vi "Conbasemela.vi"() -> ()   [LabVIEW 2020]
uses:
  PAGINAS.ctl
  <vilib>/Utility/NIReport.llb/Report Type.ctl
  <vilib>/addons/_office/excel.llb/Excel Get Data ([str]).vi
  <vilib>/Utility/NIReport.llb/Append Text Table to Report (wrap).vi
  <vilib>/regexp/Match Regular Expression.xnode
  <vilib>/Utility/NIReport.llb/NI_report.lvclass
  <vilib>/Utility/NIReport.llb/Excel/NI_Excel.lvclass
  <vilib>/Utility/NIReport.llb/NI_ReportGenerationCore.lvlib
  <vilib>/addons/_office/NI_ReportGenerationToolkit.lvlib
panel:
  in  "Sesion Iniciada TAB2":string[](array[string])
  in  "Sesion Iniciada TAB1":string[](array[string])
  in  "Tab Control 2":enum32{"LOGIN", "ADMIN", "USUARIO"}(tab)
  in  "INGRESAR 2":bool
  in  "Usuario 2":string
  in  "Contraseña 2":string
  in  "Pass add/elim 2":string
  in  "User add/elim 2":string
  in  "Terminar sesion admin 2":bool=TRUE
  in  "Añadir usuario 2":bool=TRUE
  in  "Eliminar usuario 2":bool=TRUE
  out "Dados de alta 2":string[](array[string])
  in  "Terminar sesion 2":bool=TRUE
  out "String 2":string="Hola"
  in  "MS Office parameters 2":T1={"position (excel)"={"row"=0, "column"=1}, "name (excel)"="", "bookmark (word)"=""}
  in  "MS Office parameters":T1={"position (excel)"={"row"=0, "column"=1}, "name (excel)"="", "bookmark (word)"=""}
  out "usupass juntos":string[][](array[string])
  out "data":string[][](array[string])
  in  "Pass":string[](array[string])
  in  "Usu":string[](array[string])
  in  "Tab Control":enum32{"LOGIN", "ADMIN", "USUARIO"}(tab)
  in  "INGRESAR":bool
  in  "Usuario":string
  in  "Contraseña":string
  in  "Pass add/elim":string
  in  "User add/elim":string
  in  "Terminar sesion admin":bool=TRUE
  in  "Añadir usuario":bool=TRUE
  in  "Eliminar usuario":bool=TRUE
  out "Dados de alta":string[](array[string])
  in  "Terminar sesion":bool=TRUE
  out "String":string="Hola"
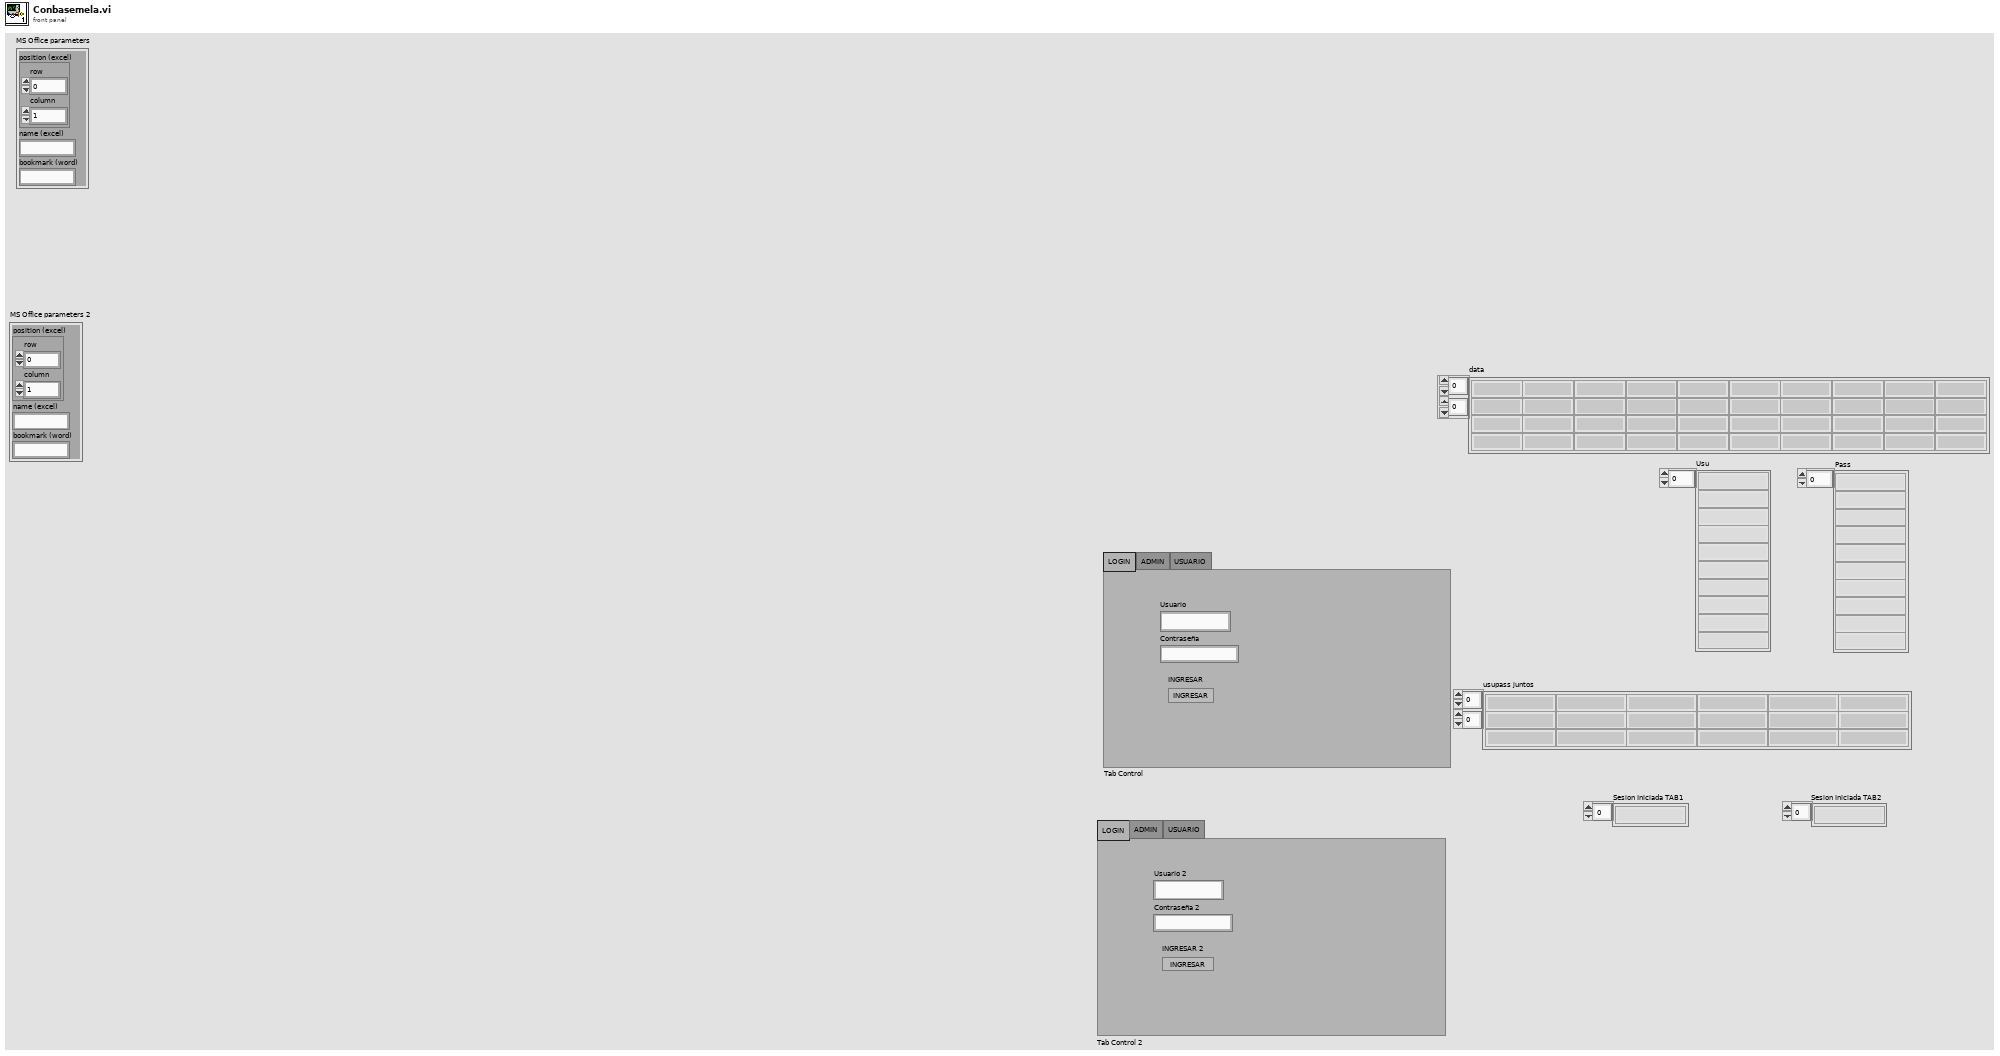
[diagram p1: front panel]
types:
  T1 = cluster{"position (excel)":cluster{"row":i32, "column":i32}, "name (excel)":string, "bookmark (word)":string}
  T2 = typedef "PAGINAS.ctl" = enum16{"0", "1", "2", "3"}
  T3 = typedef "NI_ReportGenerationCore.lvlib/Report Type.ctl" = enum16{"HTML", "Word", "Excel"}
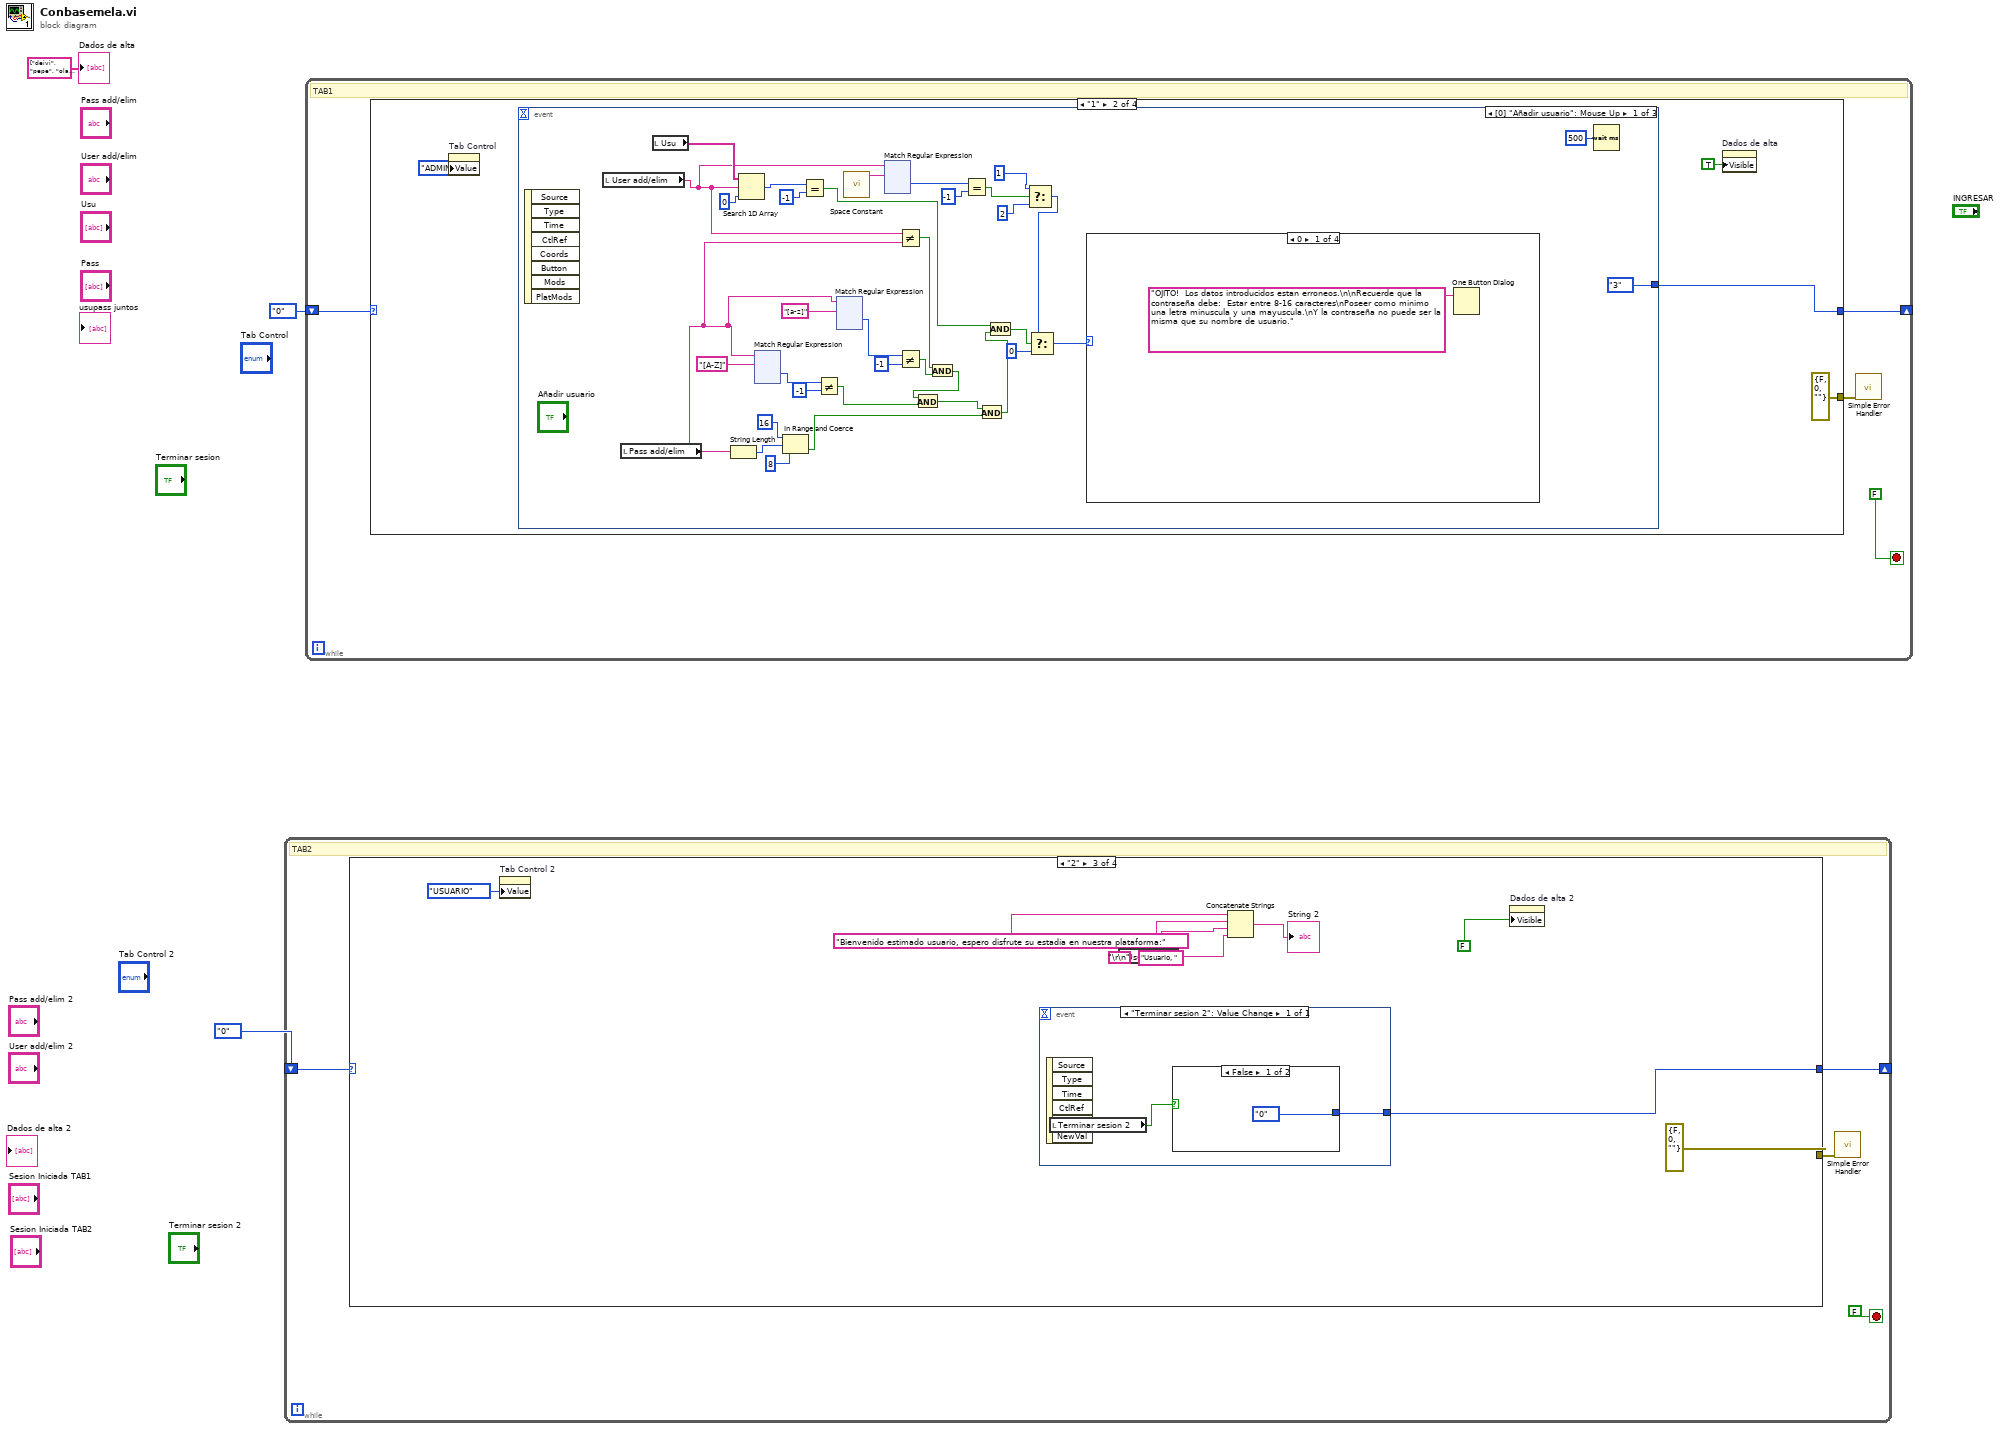
[diagram p0: block diagram]
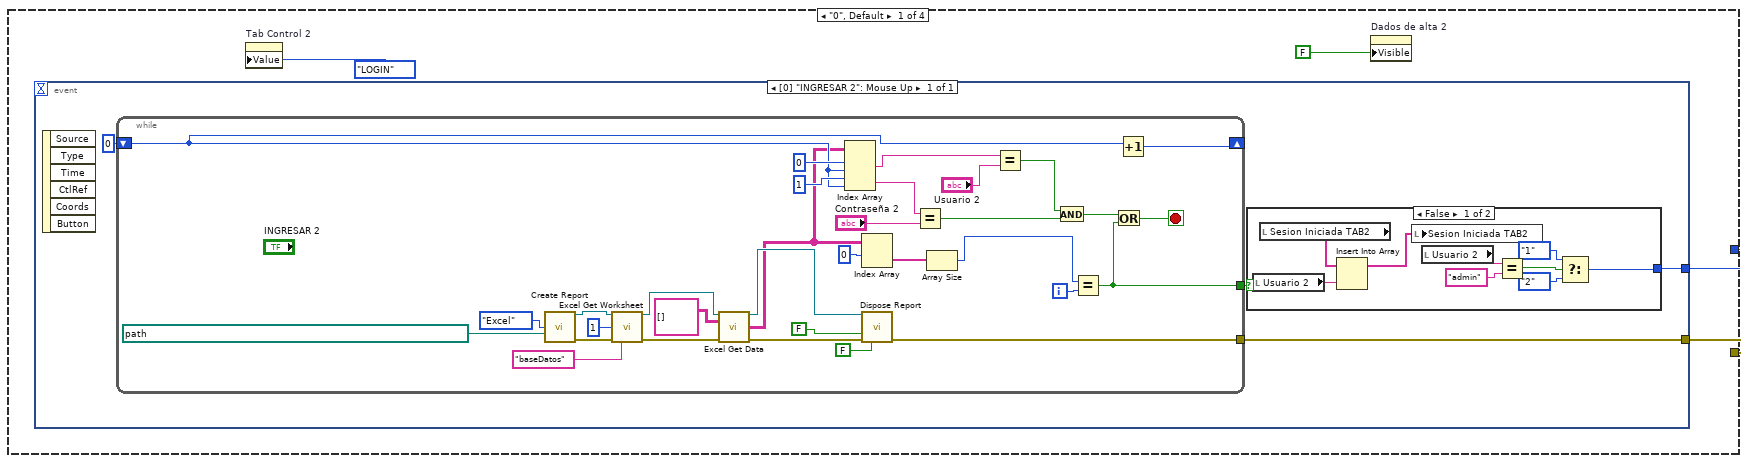
[diagram p2: hidden frame]
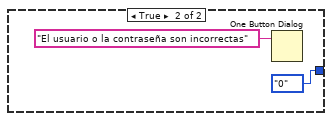
[diagram p3: hidden frame]
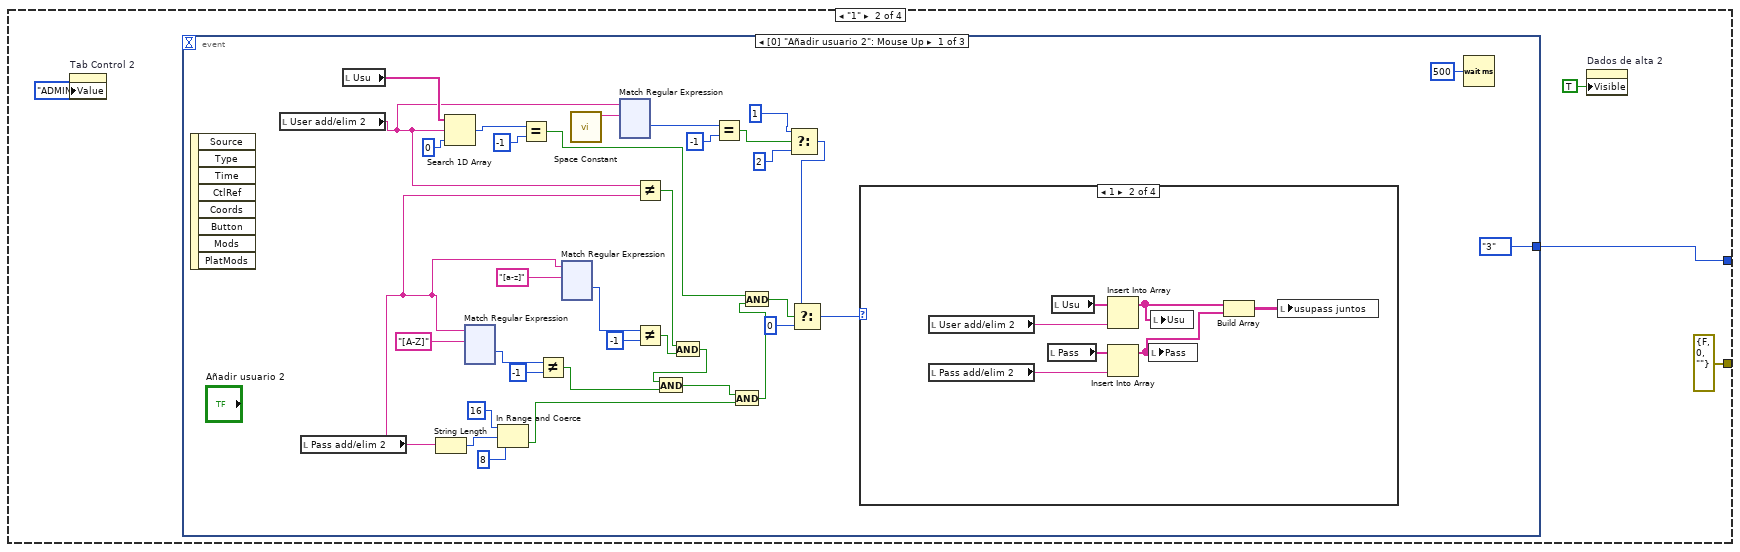
[diagram p4: hidden frame]
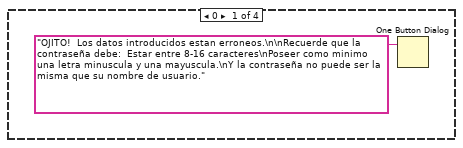
[diagram p5: hidden frame]
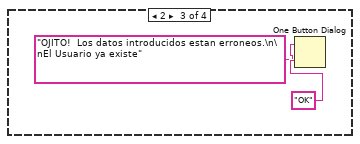
[diagram p6: hidden frame]
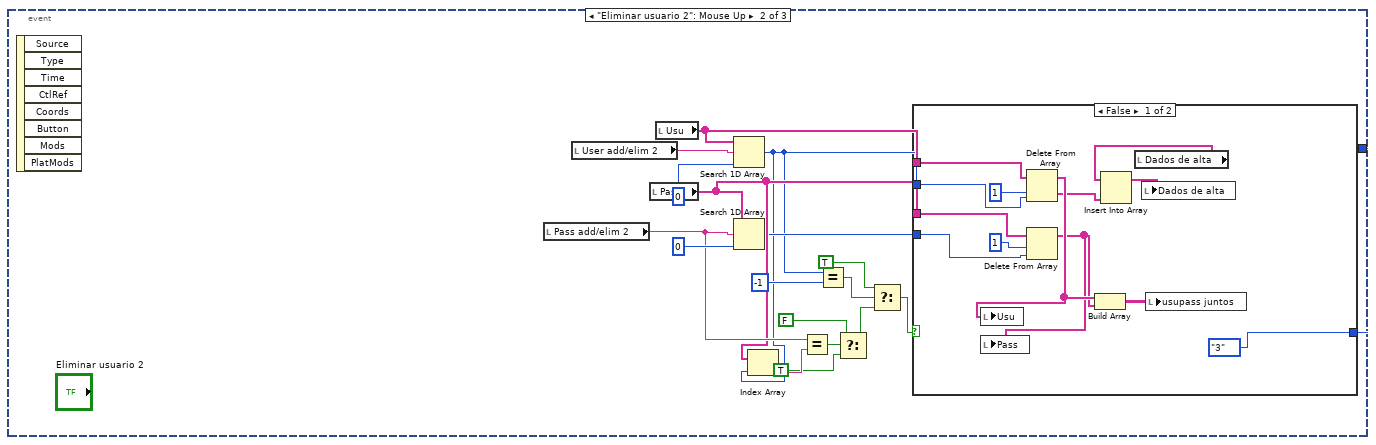
[diagram p8: hidden frame]
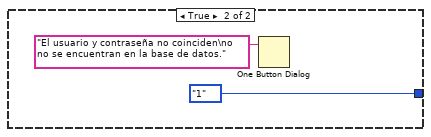
[diagram p9: hidden frame]
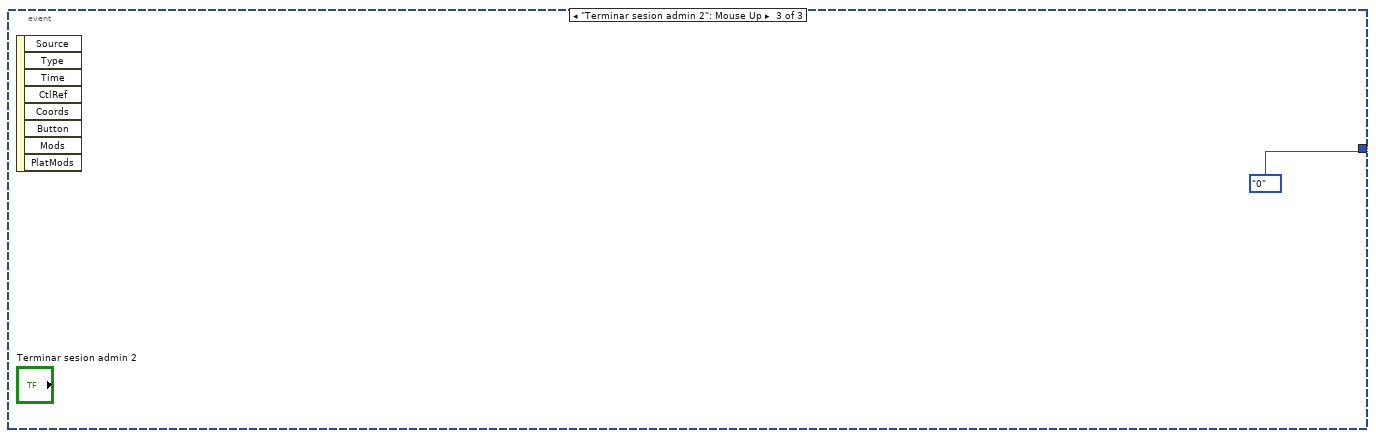
[diagram p10: hidden frame]
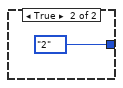
[diagram p11: hidden frame]
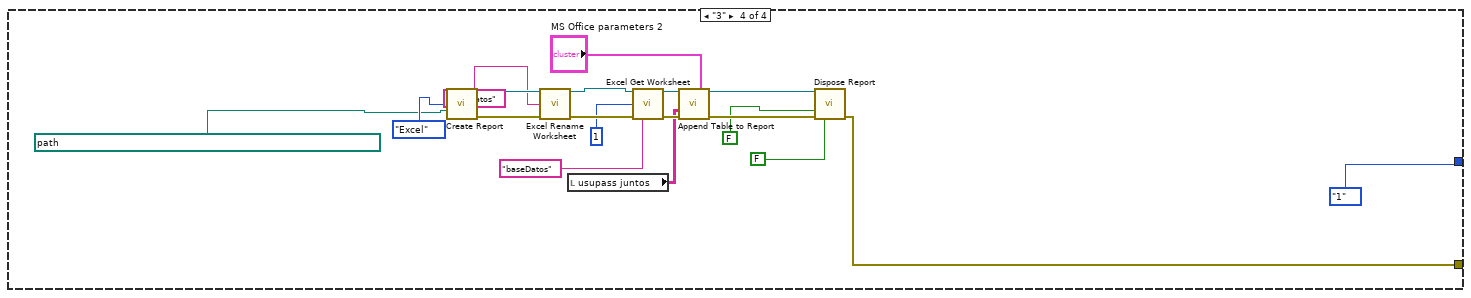
[diagram p12: hidden frame]
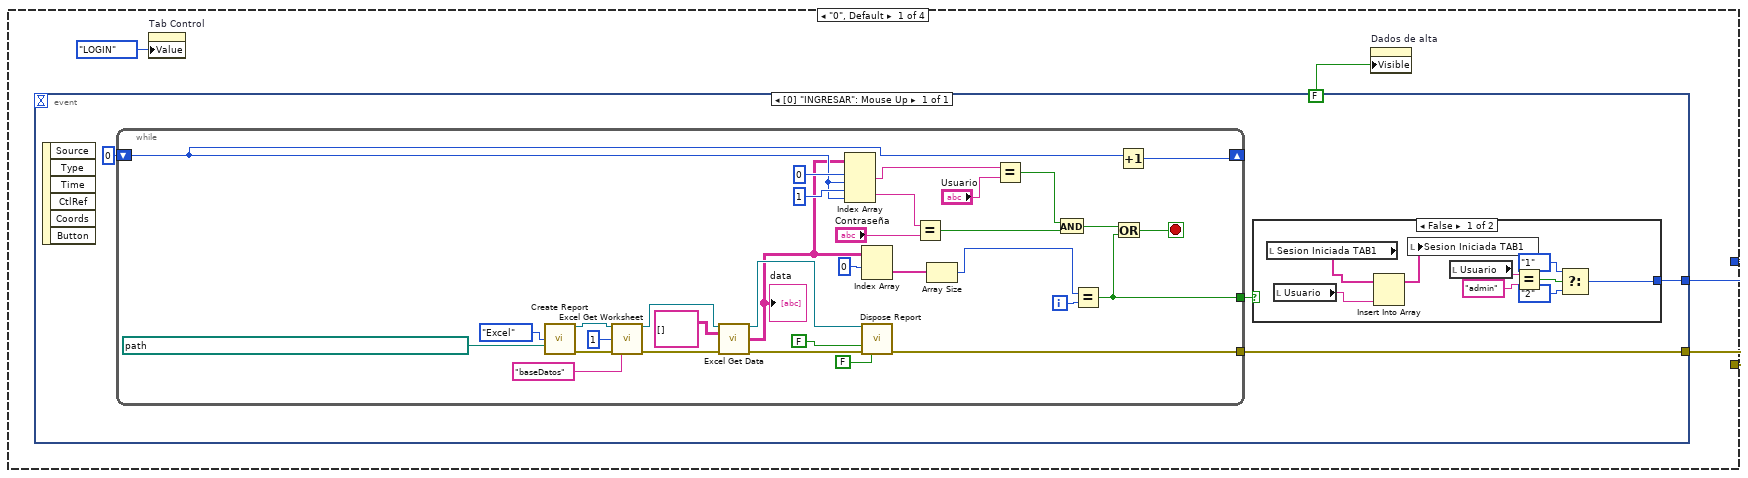
[diagram p13: hidden frame]
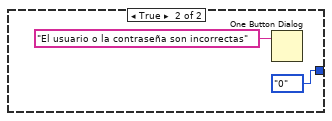
[diagram p14: hidden frame]
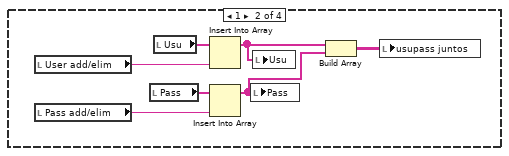
[diagram p15: hidden frame]
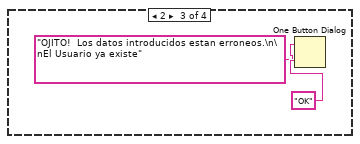
[diagram p16: hidden frame]
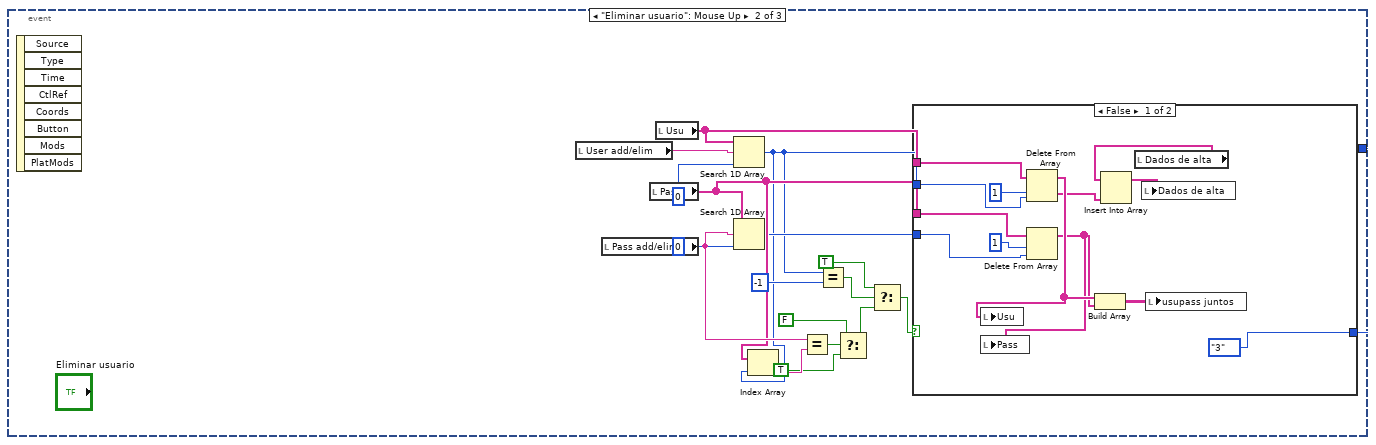
[diagram p18: hidden frame]
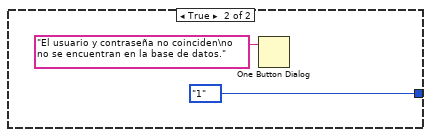
[diagram p19: hidden frame]
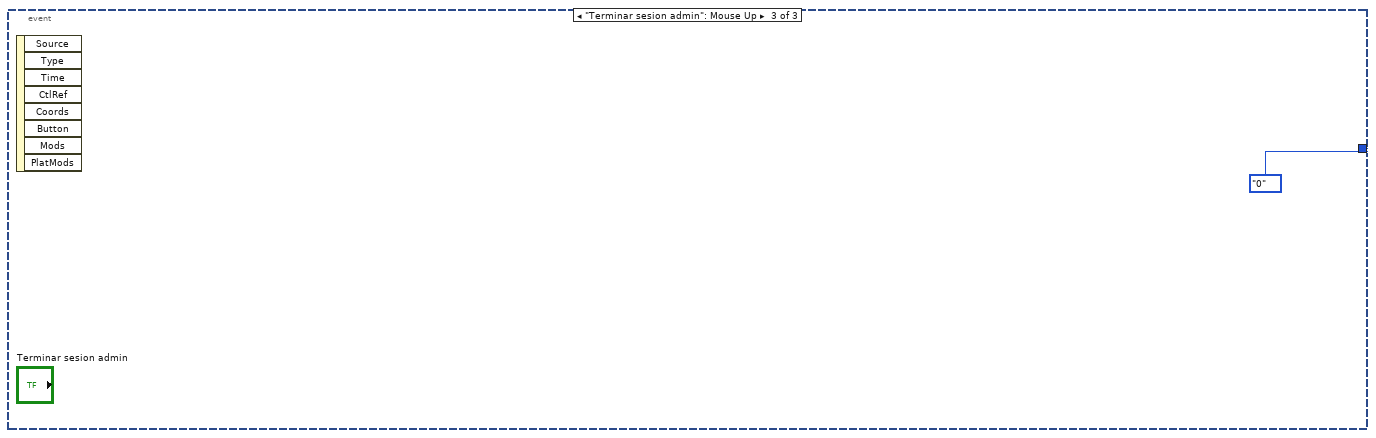
[diagram p20: hidden frame]
diagram:
  n1 = while {
    shift-right: [w6] -> _
    shift-left: PAGINAS."0" ("Enum") -> [w7]
    stop <- FALSE stop-if-true
    # "TAB2"
    n2 = case shown="\"2\"" w7 {
      tunnel: [w10 w61 w484 PAGINAS."1" ("Enum")] -> w6
      tunnel: [w9 errorcluster {"status"=FALSE, "code"=0, "source"=""} ("error out") errorcluster {"status"=FALSE, "code"=0, "source"=""} ("error out") w498] -> w4
      frame "0", Default {
        n3 = event shown="[0] \"INGRESAR 2\": Mouse Up" {
          selector: _ -> [_]
          dyn-events: _ -> [_]
          timeout: _ -> [_]
          tunnel: [w13] -> w10
          tunnel: [w12] -> w9
          event "INGRESAR 2": Mouse Up {
            n4 = event-data() -> ()  [unwired: 1 in, 6 out]
            n5 = while {
              shift-right: [w46] -> _
              shift-left: 0 -> [w39]
              tunnel: [w28] -> w14
              tunnel: [w27] -> w12
              i -> [w32]
              stop <- w29 stop-if-true
              n6 = call <vilib>:"Create Report.vi"("report type"=Report_Type."Excel", "template (empty)"=path "E:/2020-2/Lenguaje de programación ll/quiz 3.1/baseDatos.xlsx" ("file path (dialog if empty)")) -> ("report out"=w56:refnum<class "NI_report.lvclass">, "error out"=w55:errorcluster)  [unwired: 12 in]
              n7 = call <vilib>:"Excel Get Worksheet.vi"("report in"=w56, "worksheet index (0)"=1, "error in (no error)"=w55, "name (\"\")"="baseDatos" ("name (\"\")")) -> ("report out"=w53:refnum<class "NI_report.lvclass">, "error out"=w52:errorcluster)  [unwired: 10 in]
              n8 = call-poly <vilib>:"Excel Get Data.vi"("report in"=w53, "data type"=string[][] [], "error in (no error)"=w52) -> ("report out"=w51:refnum<class "NI_report.lvclass">, "data"=w35:string[][], "error out"=w50:errorcluster)  [unwired: 10 in]
              n9 = Index Array(array=w35, index (row) #1=0 ("index (row)"), index (col) #1=w39, index (row) #2=1 ("index (row)"), index (col) #2=w39) -> (element #1=w45:string, element #2=w38:string)
              n10 = Index Array(array=w35, index (row)=0) -> (element=w33:string[])  [unwired: 1 in]
              n11 = call-dynamic "Dispose Report.vi"("report in"=w51, "save changes? (F)"=FALSE, "error in (no error)"=w50, "close report? (T)"=FALSE) -> ("error out"=w27:errorcluster)  [unwired: 11 in]
              n12 = Equal?(x=w38, y="Contraseña 2") -> (x = y?=w42:bool)
              n13 = Array Size(array=w33) -> (size(s)=w31:i32)
              n14 = Equal?(x=w45, y="Usuario 2") -> (x = y?=w43:bool)
              n15 = And(x=w43, y=w42) -> (x .and. y?=w30:bool)
              n16 = Equal?(x=w31, y=w32) -> (x = y?=w28:bool)
              n17 = Or(x=w30, y=w28) -> (x .or. y?=w29:bool)
              n18 = Increment(x=w39) -> (x+1=w46:i32)
            }
            n19 = case shown="False" w14 {
              tunnel: [w19 PAGINAS."0" ("Enum")] -> w13
              frame False {
                n20 = local read "Usuario 2"() -> (w18:string)
                n21 = local read "Sesion Iniciada TAB2"() -> (w16:string[])
                n22 = Insert Into Array(array=w16, new element=w18) -> (w17:string[])  [unwired: 1 in]
                n23 = local write "Sesion Iniciada TAB2"(w17) -> ()
                n24 = local read "Usuario 2"() -> (w23:string)
                n25 = Equal?(x=w23, y="admin") -> (x = y?=w24:bool)
                n26 = Select(t=PAGINAS."1" ("Enum"), s=w24, f=PAGINAS."2" ("Enum")) -> (s? t:f=w19:T2)
              }
              frame True {
                n27 = One Button Dialog(message="El usuario o la contraseña son incorrectas") -> ()  [unwired: 1 in, 1 out]
              }
            }
          }
        }
        n28 = property on="Tab Control 2" class="TabCtl (strict)"("Value"=enum32{"LOGIN", "ADMIN", "USUARIO"}."LOGIN" ("Tab Control")) -> ()  [unwired: 2 in, 2 out]
        n29 = property on="Dados de alta 2" class="Arr (strict)"("Visible"=FALSE) -> ()  [unwired: 2 in, 2 out]
      }
      frame "1" {
        n30 = property on="Tab Control 2" class="TabCtl (strict)"("Value"=enum32{"LOGIN", "ADMIN", "USUARIO"}."ADMIN" ("Tab Control")) -> ()  [unwired: 2 in, 2 out]
        n31 = event shown="[0] \"Añadir usuario 2\": Mouse Up" {
          selector: _ -> [_ _ _]
          dyn-events: _ -> [_ _ _]
          timeout: _ -> [_ _ _]
          tunnel: [PAGINAS."3" ("Enum") w463 PAGINAS."0" ("Enum")] -> w61
          event "Añadir usuario 2": Mouse Up {
            n32 = event-data() -> ()  [unwired: 1 in, 8 out]
            n33 = local read "User add/elim 2"() -> (w75:string)
            n34 = local read "Pass add/elim 2"() -> (w79:string)
            n35 = local read "Usu"() -> (w96:string[])
            n36 = String Length(string=w79) -> (length=w92:i32)
            n37 = Search 1D Array(1D array=w96, element=w75, start index (0)=0) -> (index of element=w94:i32)
            n38 = xnode "Match Regular Expression"("input string"=w79, "regular expression"="[A-Z]") -> ("offset past match"=w88:i32)  [unwired: 4 in, 4 out]
            n39 = In Range and Coerce(upper limit=16, x=w92, lower limit=8) -> (In Range?=w77:bool)  [unwired: 1 out]
            n40 = Equal?(x=w94, y=-1) -> (x = y?=w71:bool)
            n41 = Not Equal?(x=w88, y=-1) -> (x != y?=w80:bool)
            n42 = xnode "Match Regular Expression"("input string"=w79, "regular expression"="[a-z]") -> ("offset past match"=w84:i32)  [unwired: 4 in, 4 out]
            n43 = call <vilib>:"Space Constant.vi"() -> ("String"=w74:string)
            n44 = xnode "Match Regular Expression"("input string"=w75, "regular expression"=w74) -> ("offset past match"=w72:i32)  [unwired: 4 in, 4 out]
            n45 = Not Equal?(x=w75, y=w79) -> (x != y?=w78:bool)
            n46 = Not Equal?(x=w84, y=-1) -> (x != y?=w82:bool)
            n47 = And(x=w78, y=w82) -> (x .and. y?=w81:bool)
            n48 = And(x=w81, y=w80) -> (x .and. y?=w76:bool)
            n49 = Equal?(x=w72, y=-1) -> (x = y?=w69:bool)
            n50 = And(x=w76, y=w77) -> (x .and. y?=w70:bool)
            n51 = And(x=w71, y=w70) -> (x .and. y?=w67:bool)
            n52 = Select(t=1 ("y"), s=w69, f=2 ("y")) -> (s? t:f=w66:i32)
            n53 = Select(t=w66, s=w67, f=0) -> (s? t:f=w65:i32)
            n54 = case shown="1" w65 {
              frame 0 {
                n55 = One Button Dialog(message="OJITO!  Los datos introducidos estan erroneos.\n\nRecuerde que la contraseña debe:  Estar entre 8-16 caracteres\nPoseer como minimo una letra minuscula y una mayuscula.\nY la contraseña no puede ser la misma que su nombre de usuario.") -> ()  [unwired: 1 in, 1 out]
              }
              frame 1 {
                n56 = local read "User add/elim 2"() -> (w216:string)
                n57 = local read "Pass add/elim 2"() -> (w217:string)
                n58 = local read "Pass"() -> (w218:string[])
                n59 = local read "Usu"() -> (w219:string[])
                n60 = Insert Into Array(array=w219, new element=w216) -> (w215:string[])  [unwired: 1 in]
                n61 = Insert Into Array(array=w218, new element=w217) -> (w214:string[])  [unwired: 1 in]
                n62 = local write "Pass"(w214) -> ()
                n63 = local write "Usu"(w215) -> ()
                n64 = Build Array(w215, w214) -> (w213:string[][])
                n65 = local write "usupass juntos"(w213) -> ()
              }
              frame 2 {
                n66 = One Button Dialog(message="OJITO!  Los datos introducidos estan erroneos.\n\nEl Usuario ya existe", button name ("OK")="OK") -> ()  [unwired: 1 out]
              }
              frame 3, Default {
              }
            }
            n67 = Wait (ms)(milliseconds to wait=u32 500) -> ()  [unwired: 1 out]
          }
          event "Eliminar usuario 2": Mouse Up {
            n68 = event-data() -> ()  [unwired: 1 in, 8 out]
            n69 = local read "Pass add/elim 2"() -> (w461:string)
            n70 = local read "User add/elim 2"() -> (w467:string)
            n71 = local read "Pass"() -> (w453:string[])
            n72 = local read "Usu"() -> (w451:string[])
            n73 = Search 1D Array(1D array=w451, element=w467, start index (0)=0) -> (index of element=w450:i32)
            n74 = Search 1D Array(1D array=w453, element=w461, start index (0)=0) -> (index of element=w452:i32)
            n75 = Index Array(array=w453, index=w450) -> (element=w462:string)
            n76 = Equal?(x=w461, y=w462) -> (x = y?=w457:bool)
            n77 = Equal?(x=w450, y=-1) -> (x = y?=w460:bool)
            n78 = Select(t=FALSE, s=w457, f=TRUE) -> (s? t:f=w454:bool)
            n79 = Select(t=TRUE, s=w460, f=w454) -> (s? t:f=w458:bool)
            n80 = case shown="False" w458 {
              tunnel: [PAGINAS."3" ("Enum") PAGINAS."1" ("Enum")] -> w463
              tunnel: w453 -> [w479 _]
              tunnel: w452 -> [w477 _]
              tunnel: w451 -> [w476 _]
              tunnel: w450 -> [w474 _]
              frame False {
                n81 = Delete From Array(array=w476, length=1, index=w474) -> (deleted portion=w469:string[], array with subset deleted=w472:string[])
                n82 = local write "Usu"(w472) -> ()
                n83 = Delete From Array(array=w479, length=1, index=w477) -> (array with subset deleted=w471:string[])  [unwired: 1 out]
                n84 = local write "Pass"(w471) -> ()
                n85 = Build Array(w472, w471) -> (w473:string[][])
                n86 = local read "Dados de alta"() -> (w470:string[])
                n87 = Insert Into Array(array=w470, new element=w469) -> (w468:string[])  [unwired: 1 in]
                n88 = local write "Dados de alta"(w468) -> ()
                n89 = local write "usupass juntos"(w473) -> ()
              }
              frame True {
                n90 = One Button Dialog(message="El usuario y contraseña no coinciden\no no se encuentran en la base de datos.") -> ()  [unwired: 1 in, 1 out]
              }
            }
          }
          event "Terminar sesion admin 2": Mouse Up {
            n91 = event-data() -> ()  [unwired: 1 in, 8 out]
          }
        }
        n92 = property on="Dados de alta 2" class="Arr (strict)"("Visible"=TRUE) -> ()  [unwired: 2 in, 2 out]
      }
      frame "2" {
        n93 = property on="Tab Control 2" class="TabCtl (strict)"("Value"=enum32{"LOGIN", "ADMIN", "USUARIO"}."USUARIO" ("Tab Control")) -> ()  [unwired: 2 in, 2 out]
        n94 = event shown="[0] \"Terminar sesion 2\": Value Change" {
          selector: _ -> [_]
          dyn-events: _ -> [_]
          timeout: _ -> [_]
          tunnel: [w493] -> w484
          event "Terminar sesion 2": Value Change {
            n95 = event-data() -> ()  [unwired: 1 in, 6 out]
            n96 = local read "Terminar sesion 2"() -> (w494:bool)
            n97 = case shown="False" w494 {
              tunnel: [PAGINAS."0" ("Enum") PAGINAS."2" ("Enum")] -> w493
              frame False {
              }
              frame True {
              }
            }
          }
        }
        n98 = local read "Usuario 2"() -> (w486:string)
        n99 = Concatenate Strings("Bienvenido estimado usuario, espero disfrute su estadía en nuestra plataforma:" ("string"), "\r\n", "Usuario, " ("string"), w486) -> (→"String 2":string)
        n100 = property on="Dados de alta 2" class="Arr (strict)"("Visible"=FALSE) -> ()  [unwired: 2 in, 2 out]
      }
      frame "3" {
        n101 = call <vilib>:"Create Report.vi"("report type"=Report_Type."Excel", "template (empty)"=path "E:/2020-2/Lenguaje de programación ll/quiz 3.1/baseDatos.xlsx" ("file path (dialog if empty)")) -> ("report out"=w513:refnum<class "NI_report.lvclass">, "error out"=w514:errorcluster)  [unwired: 12 in]
        n102 = call <vilib>:"Excel Rename Worksheet.vi"("report in"=w513, "worksheet name (\"\")"="baseDatos" ("worksheet name (\"\")"), "error in (no error)"=w514) -> ("report out"=w512:refnum<class "NI_report.lvclass">, "error out"=w515:errorcluster)  [unwired: 11 in]
        n103 = local read "usupass juntos"() -> (w497:string[][])
        n104 = call <vilib>:"Excel Get Worksheet.vi"("report in"=w512, "worksheet index (0)"=1, "error in (no error)"=w515, "name (\"\")"="baseDatos" ("name (\"\")")) -> ("report out"=w510:refnum<class "NI_report.lvclass">, "error out"=w509:errorcluster)  [unwired: 10 in]
        n105 = call-poly <vilib>:"Append Table to Report.vi"("report in"=w510, "MS Office parameters"="MS Office parameters 2", "text data"=w497, "error in (no error)"=w509) -> ("report out"=w508:refnum<class "NI_report.lvclass">, "error out"=w507:errorcluster)  [unwired: 8 in, 2 out]
        n106 = call-dynamic "Dispose Report.vi"("report in"=w508, "save changes? (F)"=FALSE, "error in (no error)"=w507, "close report? (T)"=FALSE) -> ("error out"=w498:errorcluster)  [unwired: 11 in]
      }
    }
    n107 = call <vilib>:"Simple Error Handler.vi"("error in (no error)"=w4) -> ()  [unwired: 4 in, 5 out]
  }
  n108 = while {
    shift-right: [w518] -> _
    shift-left: PAGINAS."0" ("Enum") -> [w519]
    stop <- FALSE stop-if-true
    # "TAB1"
    n109 = case shown="\"1\"" w519 {
      tunnel: [w522 w573 w996 PAGINAS."1" ("Enum")] -> w518
      tunnel: [w521 errorcluster {"status"=FALSE, "code"=0, "source"=""} ("error out") errorcluster {"status"=FALSE, "code"=0, "source"=""} ("error out") w1010] -> w516
      frame "0", Default {
        n110 = event shown="[0] \"INGRESAR\": Mouse Up" {
          selector: _ -> [_]
          dyn-events: _ -> [_]
          timeout: _ -> [_]
          tunnel: [w525] -> w522
          tunnel: [w524] -> w521
          event "INGRESAR": Mouse Up {
            n111 = event-data() -> ()  [unwired: 1 in, 6 out]
            n112 = while {
              shift-right: [w558] -> _
              shift-left: 0 -> [w551]
              tunnel: [w540] -> w526
              tunnel: [w539] -> w524
              i -> [w544]
              stop <- w541 stop-if-true
              n113 = call <vilib>:"Create Report.vi"("report type"=Report_Type."Excel", "template (empty)"=path "E:/2020-2/Lenguaje de programación ll/quiz 3.1/baseDatos.xlsx" ("file path (dialog if empty)")) -> ("report out"=w568:refnum<class "NI_report.lvclass">, "error out"=w567:errorcluster)  [unwired: 12 in]
              n114 = call <vilib>:"Excel Get Worksheet.vi"("report in"=w568, "worksheet index (0)"=1, "error in (no error)"=w567, "name (\"\")"="baseDatos" ("name (\"\")")) -> ("report out"=w565:refnum<class "NI_report.lvclass">, "error out"=w564:errorcluster)  [unwired: 10 in]
              n115 = call-poly <vilib>:"Excel Get Data.vi"("report in"=w565, "data type"=string[][] [], "error in (no error)"=w564) -> ("report out"=w563:refnum<class "NI_report.lvclass">, "data"=w547:string[][], "error out"=w562:errorcluster)  [unwired: 10 in]
              "data" <- w547
              n116 = Index Array(array=w547, index (row) #1=0 ("index (row)"), index (col) #1=w551, index (row) #2=1 ("index (row)"), index (col) #2=w551) -> (element #1=w557:string, element #2=w550:string)
              n117 = Index Array(array=w547, index (row)=0) -> (element=w545:string[])  [unwired: 1 in]
              n118 = call-dynamic "Dispose Report.vi"("report in"=w563, "save changes? (F)"=FALSE, "error in (no error)"=w562, "close report? (T)"=FALSE) -> ("error out"=w539:errorcluster)  [unwired: 11 in]
              n119 = Equal?(x=w550, y="Contraseña") -> (x = y?=w554:bool)
              n120 = Array Size(array=w545) -> (size(s)=w543:i32)
              n121 = Equal?(x=w557, y="Usuario") -> (x = y?=w555:bool)
              n122 = And(x=w555, y=w554) -> (x .and. y?=w542:bool)
              n123 = Equal?(x=w543, y=w544) -> (x = y?=w540:bool)
              n124 = Or(x=w542, y=w540) -> (x .or. y?=w541:bool)
              n125 = Increment(x=w551) -> (x+1=w558:i32)
            }
            n126 = case shown="False" w526 {
              tunnel: [w531 PAGINAS."0" ("Enum")] -> w525
              frame False {
                n127 = local read "Sesion Iniciada TAB1"() -> (w530:string[])
                n128 = local read "Usuario"() -> (w529:string)
                n129 = Insert Into Array(array=w530, new element=w529) -> (w528:string[])  [unwired: 1 in]
                n130 = local write "Sesion Iniciada TAB1"(w528) -> ()
                n131 = local read "Usuario"() -> (w535:string)
                n132 = Equal?(x=w535, y="admin") -> (x = y?=w536:bool)
                n133 = Select(t=PAGINAS."1" ("Enum"), s=w536, f=PAGINAS."2" ("Enum")) -> (s? t:f=w531:T2)
              }
              frame True {
                n134 = One Button Dialog(message="El usuario o la contraseña son incorrectas") -> ()  [unwired: 1 in, 1 out]
              }
            }
          }
        }
        n135 = property on="Tab Control" class="TabCtl (strict)"("Value"=enum32{"LOGIN", "ADMIN", "USUARIO"}."LOGIN" ("Tab Control")) -> ()  [unwired: 2 in, 2 out]
        n136 = property on="Dados de alta" class="Arr (strict)"("Visible"=FALSE) -> ()  [unwired: 2 in, 2 out]
      }
      frame "1" {
        n137 = property on="Tab Control" class="TabCtl (strict)"("Value"=enum32{"LOGIN", "ADMIN", "USUARIO"}."ADMIN" ("Tab Control")) -> ()  [unwired: 2 in, 2 out]
        n138 = event shown="[0] \"Añadir usuario\": Mouse Up" {
          selector: _ -> [_ _ _]
          dyn-events: _ -> [_ _ _]
          timeout: _ -> [_ _ _]
          tunnel: [PAGINAS."3" ("Enum") w975 PAGINAS."0" ("Enum")] -> w573
          event "Añadir usuario": Mouse Up {
            n139 = event-data() -> ()  [unwired: 1 in, 8 out]
            n140 = local read "User add/elim"() -> (w587:string)
            n141 = local read "Pass add/elim"() -> (w591:string)
            n142 = local read "Usu"() -> (w608:string[])
            n143 = String Length(string=w591) -> (length=w604:i32)
            n144 = Search 1D Array(1D array=w608, element=w587, start index (0)=0) -> (index of element=w606:i32)
            n145 = xnode "Match Regular Expression"("input string"=w591, "regular expression"="[A-Z]") -> ("offset past match"=w600:i32)  [unwired: 4 in, 4 out]
            n146 = In Range and Coerce(upper limit=16, x=w604, lower limit=8) -> (In Range?=w589:bool)  [unwired: 1 out]
            n147 = Equal?(x=w606, y=-1) -> (x = y?=w583:bool)
            n148 = Not Equal?(x=w600, y=-1) -> (x != y?=w592:bool)
            n149 = xnode "Match Regular Expression"("input string"=w591, "regular expression"="[a-z]") -> ("offset past match"=w596:i32)  [unwired: 4 in, 4 out]
            n150 = call <vilib>:"Space Constant.vi"() -> ("String"=w586:string)
            n151 = xnode "Match Regular Expression"("input string"=w587, "regular expression"=w586) -> ("offset past match"=w584:i32)  [unwired: 4 in, 4 out]
            n152 = Not Equal?(x=w587, y=w591) -> (x != y?=w590:bool)
            n153 = Not Equal?(x=w596, y=-1) -> (x != y?=w594:bool)
            n154 = And(x=w590, y=w594) -> (x .and. y?=w593:bool)
            n155 = And(x=w593, y=w592) -> (x .and. y?=w588:bool)
            n156 = Equal?(x=w584, y=-1) -> (x = y?=w581:bool)
            n157 = And(x=w588, y=w589) -> (x .and. y?=w582:bool)
            n158 = And(x=w583, y=w582) -> (x .and. y?=w579:bool)
            n159 = Select(t=1 ("y"), s=w581, f=2 ("y")) -> (s? t:f=w578:i32)
            n160 = Select(t=w578, s=w579, f=0) -> (s? t:f=w577:i32)
            n161 = case shown="0" w577 {
              frame 0 {
                n162 = One Button Dialog(message="OJITO!  Los datos introducidos estan erroneos.\n\nRecuerde que la contraseña debe:  Estar entre 8-16 caracteres\nPoseer como minimo una letra minuscula y una mayuscula.\nY la contraseña no puede ser la misma que su nombre de usuario.") -> ()  [unwired: 1 in, 1 out]
              }
              frame 1 {
                n163 = local read "User add/elim"() -> (w728:string)
                n164 = local read "Pass add/elim"() -> (w729:string)
                n165 = local read "Pass"() -> (w730:string[])
                n166 = local read "Usu"() -> (w731:string[])
                n167 = Insert Into Array(array=w731, new element=w728) -> (w727:string[])  [unwired: 1 in]
                n168 = Insert Into Array(array=w730, new element=w729) -> (w726:string[])  [unwired: 1 in]
                n169 = local write "Pass"(w726) -> ()
                n170 = local write "Usu"(w727) -> ()
                n171 = Build Array(w727, w726) -> (w725:string[][])
                n172 = local write "usupass juntos"(w725) -> ()
              }
              frame 2 {
                n173 = One Button Dialog(message="OJITO!  Los datos introducidos estan erroneos.\n\nEl Usuario ya existe", button name ("OK")="OK") -> ()  [unwired: 1 out]
              }
              frame 3, Default {
              }
            }
            n174 = Wait (ms)(milliseconds to wait=u32 500) -> ()  [unwired: 1 out]
          }
          event "Eliminar usuario": Mouse Up {
            n175 = event-data() -> ()  [unwired: 1 in, 8 out]
            n176 = local read "User add/elim"() -> (w979:string)
            n177 = local read "Pass add/elim"() -> (w973:string)
            n178 = local read "Pass"() -> (w965:string[])
            n179 = local read "Usu"() -> (w963:string[])
            n180 = Search 1D Array(1D array=w963, element=w979, start index (0)=0) -> (index of element=w962:i32)
            n181 = Search 1D Array(1D array=w965, element=w973, start index (0)=0) -> (index of element=w964:i32)
            n182 = Index Array(array=w965, index=w962) -> (element=w974:string)
            n183 = Equal?(x=w973, y=w974) -> (x = y?=w969:bool)
            n184 = Equal?(x=w962, y=-1) -> (x = y?=w972:bool)
            n185 = Select(t=FALSE, s=w969, f=TRUE) -> (s? t:f=w966:bool)
            n186 = Select(t=TRUE, s=w972, f=w966) -> (s? t:f=w970:bool)
            n187 = case shown="False" w970 {
              tunnel: [PAGINAS."3" ("Enum") PAGINAS."1" ("Enum")] -> w975
              tunnel: w965 -> [w991 _]
              tunnel: w964 -> [w989 _]
              tunnel: w963 -> [w988 _]
              tunnel: w962 -> [w986 _]
              frame False {
                n188 = Delete From Array(array=w988, length=1, index=w986) -> (deleted portion=w981:string[], array with subset deleted=w984:string[])
                n189 = local write "Usu"(w984) -> ()
                n190 = Delete From Array(array=w991, length=1, index=w989) -> (array with subset deleted=w983:string[])  [unwired: 1 out]
                n191 = local write "Pass"(w983) -> ()
                n192 = Build Array(w984, w983) -> (w985:string[][])
                n193 = local read "Dados de alta"() -> (w982:string[])
                n194 = Insert Into Array(array=w982, new element=w981) -> (w980:string[])  [unwired: 1 in]
                n195 = local write "Dados de alta"(w980) -> ()
                n196 = local write "usupass juntos"(w985) -> ()
              }
              frame True {
                n197 = One Button Dialog(message="El usuario y contraseña no coinciden\no no se encuentran en la base de datos.") -> ()  [unwired: 1 in, 1 out]
              }
            }
          }
          event "Terminar sesion admin": Mouse Up {
            n198 = event-data() -> ()  [unwired: 1 in, 8 out]
          }
        }
        n199 = property on="Dados de alta" class="Arr (strict)"("Visible"=TRUE) -> ()  [unwired: 2 in, 2 out]
      }
      frame "2" {
        n200 = property on="Tab Control" class="TabCtl (strict)"("Value"=enum32{"LOGIN", "ADMIN", "USUARIO"}."USUARIO" ("Tab Control")) -> ()  [unwired: 2 in, 2 out]
        n201 = event shown="[0] \"Terminar sesion\": Mouse Up" {
          selector: _ -> [_]
          dyn-events: _ -> [_]
          timeout: _ -> [_]
          tunnel: [w1005] -> w996
          event "Terminar sesion": Mouse Up {
            n202 = event-data() -> ()  [unwired: 1 in, 8 out]
            n203 = local read "Terminar sesion"() -> (w1006:bool)
            n204 = case shown="True" w1006 {
              tunnel: [PAGINAS."0" ("Enum") PAGINAS."2" ("Enum")] -> w1005
              frame False {
              }
              frame True {
              }
            }
          }
        }
        n205 = local read "Usuario"() -> (w998:string)
        n206 = Concatenate Strings("Bienvenido estimado usuario, espero disfrute su estadía en nuestra plataforma:" ("string"), "\r\n", "Usuario, " ("string"), w998) -> (→"String":string)
        n207 = property on="Dados de alta" class="Arr (strict)"("Visible"=FALSE) -> ()  [unwired: 2 in, 2 out]
      }
      frame "3" {
        n208 = call <vilib>:"Create Report.vi"("report type"=Report_Type."Excel", "template (empty)"=path "E:/2020-2/Lenguaje de programación ll/quiz 3.1/baseDatos.xlsx" ("file path (dialog if empty)")) -> ("report out"=w1025:refnum<class "NI_report.lvclass">, "error out"=w1026:errorcluster)  [unwired: 12 in]
        n209 = call <vilib>:"Excel Rename Worksheet.vi"("report in"=w1025, "worksheet name (\"\")"="baseDatos" ("worksheet name (\"\")"), "error in (no error)"=w1026) -> ("report out"=w1024:refnum<class "NI_report.lvclass">, "error out"=w1027:errorcluster)  [unwired: 11 in]
        n210 = local read "usupass juntos"() -> (w1009:string[][])
        n211 = call <vilib>:"Excel Get Worksheet.vi"("report in"=w1024, "worksheet index (0)"=1, "error in (no error)"=w1027, "name (\"\")"="baseDatos" ("name (\"\")")) -> ("report out"=w1022:refnum<class "NI_report.lvclass">, "error out"=w1021:errorcluster)  [unwired: 10 in]
        n212 = call-poly <vilib>:"Append Table to Report.vi"("report in"=w1022, "MS Office parameters"="MS Office parameters", "text data"=w1009, "error in (no error)"=w1021) -> ("report out"=w1020:refnum<class "NI_report.lvclass">, "error out"=w1019:errorcluster)  [unwired: 8 in, 2 out]
        n213 = call-dynamic "Dispose Report.vi"("report in"=w1020, "save changes? (F)"=FALSE, "error in (no error)"=w1019, "close report? (T)"=FALSE) -> ("error out"=w1010:errorcluster)  [unwired: 11 in]
      }
    }
    n214 = call <vilib>:"Simple Error Handler.vi"("error in (no error)"=w516) -> ()  [unwired: 4 in, 5 out]
  }
  "Dados de alta" <- string[] ["deivi", "pepe", "ola", "ghgh"] ("Array")
